vi "LogAndCreateNewIfRequired.vi"(0 "EventData in":T2, 5 "LogDataIn":T1[](array[typedef]), 11 "error in (no error)":errorcluster) -> (4 "EventData out":T2, 15 "error out":errorcluster)   [LabVIEW 2021, in "Event Logger.lvlib"]
uses:
  Event Logger.lvlib
  TypeDef/EventDataCluster.ctl
  TypeDef/EventValues.ctl
  <vilib>/Utility/file.llb/Write Delimited Spreadsheet (string).vi
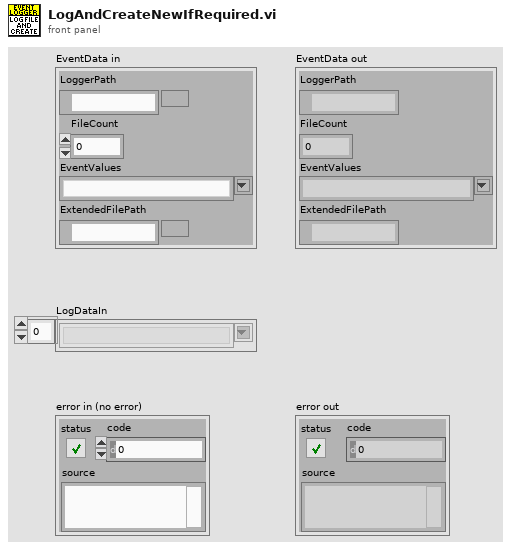
[diagram p1: front panel]
types:
  T1 = typedef "Event Logger.lvlib/EventValues.ctl" = string
  T2 = typedef "Event Logger.lvlib/EventDataCluster.ctl" = cluster{"LoggerPath":path, "FileCount":i32, "EventValues":T1, "ExtendedFilePath":path}
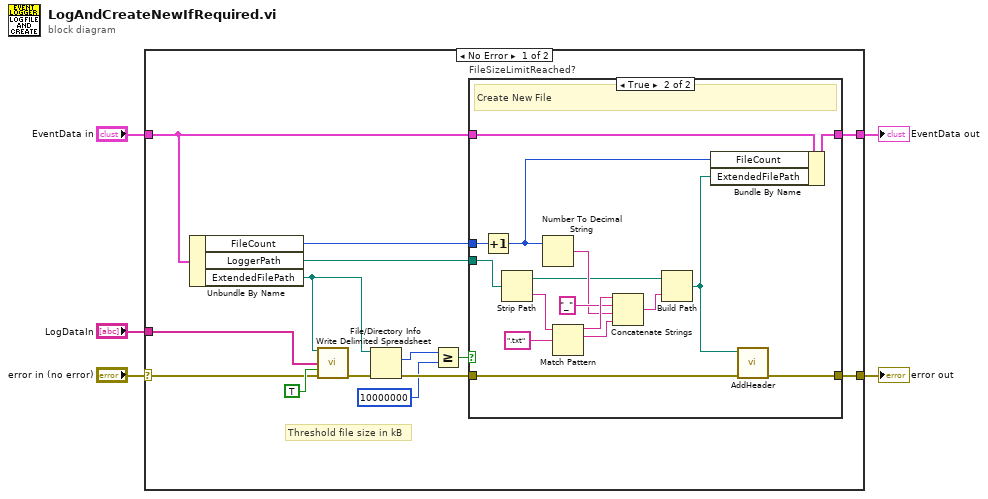
[diagram p0: block diagram]
diagram:
  n1 = case shown="No Error" "error in (no error)" {
    selector: "error in (no error)" -> [w10 w38]
    tunnel: [w19 _] -> w5
    tunnel: [w18 w38] -> w4
    tunnel: "EventData in" -> [w13 _]
    tunnel: "LogDataIn" -> [w8 _]
    frame No Error {
      # "Threshold file size in kB"
      n2 = Unbundle By Name(w13) -> ("FileCount"=w12:i32, "LoggerPath"=w6:path, "ExtendedFilePath"=w7:path)
      n3 = call-poly <vilib>:"Write Delimited Spreadsheet.vi"("file path (dialog if empty)"=w7, "1D data"=w8, "append to file? (new file:F)"=TRUE, "error in (no error)"=w10) -> ("error out"=w9:errorcluster)  [unwired: 10 in, 1 out]
      n4 = File/Directory Info(path=w7, error in=w9) -> (size=w14:i64, error out=w16:errorcluster)  [unwired: 5 out]
      n5 = Greater Or Equal?(x=w14, y=i64 10000000) -> (x >= y?=w17:bool)
      n6 = case "FileSizeLimitReached?" shown="True" w17 {
        tunnel: w16 -> [w21 w23]
        tunnel: [w21 w24] -> w18
        tunnel: w12 -> [_ w35]
        tunnel: w13 -> [w20 w28]
        tunnel: [w20 w27] -> w19
        tunnel: w6 -> [_ w22]
        frame False {
          # "Use the same file"
        }
        frame True {
          # "Create New File"
          n7 = Increment(x=w35) -> (x+1=w26:i32)
          n8 = Strip Path(path=w22) -> (stripped path=w30:path, name=w37:string)
          n9 = Number To Decimal String(number=w26) -> (decimal integer string=w32:string)  [unwired: 1 in]
          n10 = Match Pattern(string=w37, regular expression=".txt") -> (before substring=w34:string, match substring=w31:string)  [unwired: 1 in, 2 out]
          n11 = Concatenate Strings(w34, "_" ("string"), w32, w31) -> (w29:string)
          n12 = Build Path(base path=w30, name or relative path=w29) -> (appended path=w25:path)
          n13 = Bundle By Name(cluster=w28, "FileCount"=w26, "ExtendedFilePath"=w25) -> (w27:T2)
          n14 = call "AddHeader.vi"("error in (no error)"=w23, "LoggerPath"=w25) -> ("error out"=w24:errorcluster)  [unwired: 9 in]
        }
      }
    }
    frame Error {
    }
  }
  "EventData out" <- w5
  "error out" <- w4
